vi "Win Receive data.vi"() -> ()   [LabVIEW 2017]
panel:
  in  "base path":path
  out "Waveform Chart":cluster{dbl, dbl, dbl}[](graph)
  out "error out":errorcluster
  in  "stop":bool
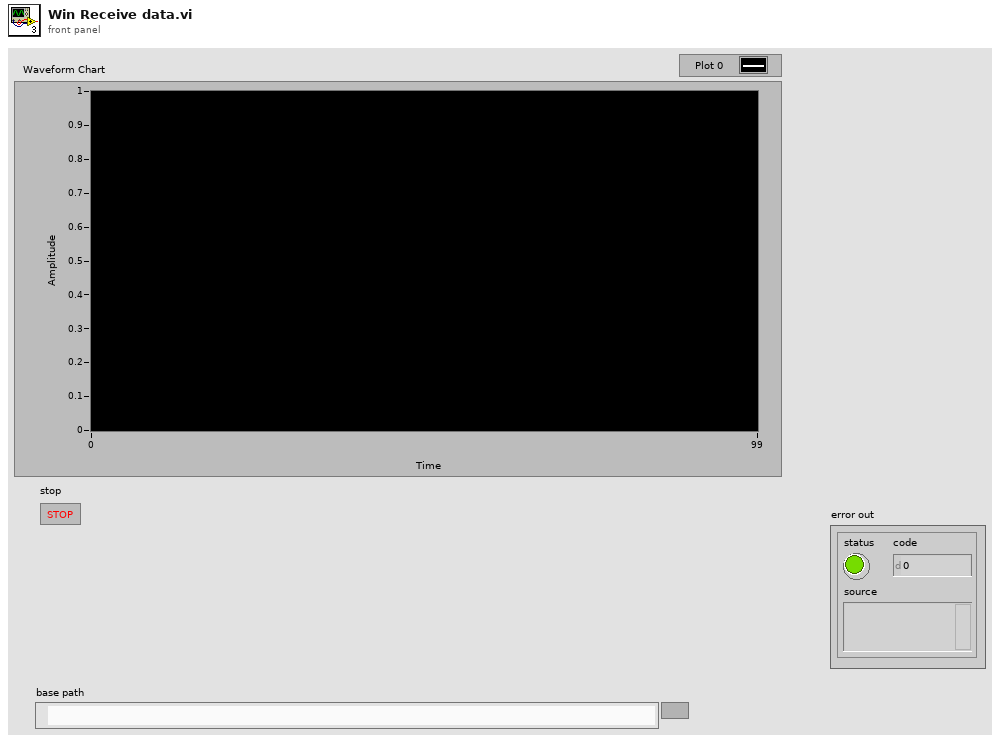
[diagram p1: front panel]
types:
  T1 = enum16{"open", "open or create", "create or replace", "create", "open (read-only)"}
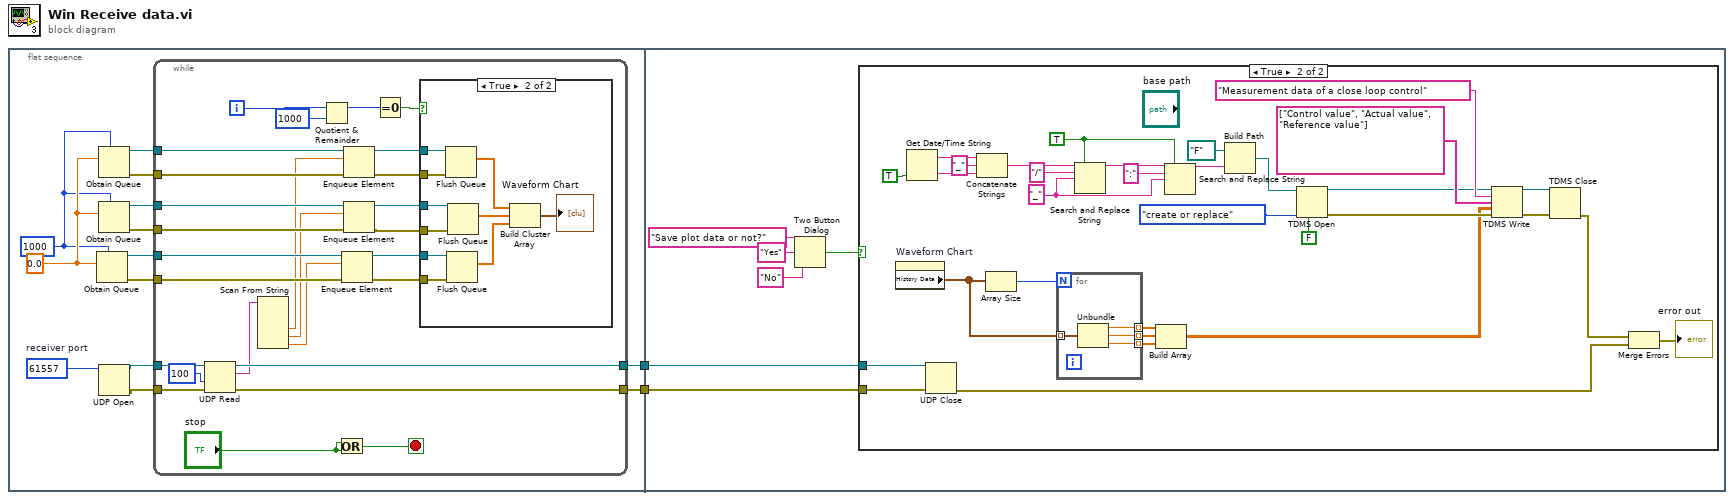
[diagram p0: block diagram]
diagram:
  n1 = flat-sequence {
    tunnel: [w4] -> w2
    tunnel: [w3] -> w1
    tunnel: w2 -> [w58]
    tunnel: w1 -> [w57]
    frame #0 {
      w12 = 0.0
      w11 = 1000 ("max queue size (-1, unlimited)")
      w15 = u16 61557  # receiver port
      n2 = Obtain Queue(max queue size (-1, unlimited)=w11, element data type=w12) -> (queue out=w6:refnum<queue>, error out=w5:errorcluster)  [unwired: 3 in, 1 out]
      n3 = Obtain Queue(max queue size (-1, unlimited)=w11, element data type=w12) -> (queue out=w10:refnum<queue>, error out=w9:errorcluster)  [unwired: 3 in, 1 out]
      n4 = Obtain Queue(max queue size (-1, unlimited)=w11, element data type=w12) -> (queue out=w8:refnum<queue>, error out=w7:errorcluster)  [unwired: 3 in, 1 out]
      n5 = UDP Open(11:w15) -> (port=w14:refnum<k16>, 0:w13:errorcluster)  [unwired: 4 in, 1 out]
      n6 = while {
        tunnel: w14 -> [w40]
        tunnel: w13 -> [w39]
        tunnel: w10 -> [w34]
        tunnel: w9 -> [w33]
        tunnel: w8 -> [w32]
        tunnel: w7 -> [w31]
        tunnel: w6 -> [w30]
        tunnel: w5 -> [w29]
        tunnel: [w22] -> w4
        tunnel: [w21] -> w3
        i -> [w36]
        stop <- w42 stop-if-true
        n7 = UDP Read(connection ID=w40, timeout ms (25000)=100 ("max size (548)"), 8:w39) -> (data out=w19:string, error out=w22:errorcluster, 3:w21:refnum<k16>)  [unwired: 3 out]
        n8 = Scan From String(input string=w19) -> (output 1=w16:dbl, output 2=w17:dbl, output 3=w18:dbl)  [unwired: 6 in, 3 out]
        n9 = Quotient & Remainder(x=w36, y=1000) -> (x-y*floor(x/y)=w37:i32)  [unwired: 1 out]
        n10 = Or(x="stop", y="stop") -> (x .or. y?=w42:bool)
        n11 = Enqueue Element(queue=w30, element=w18, error in (no error)=w29) -> (queue out=w24:refnum<queue>, error out=w23:errorcluster)  [unwired: 1 in, 1 out]
        n12 = Enqueue Element(queue=w34, element=w16, error in (no error)=w33) -> (queue out=w28:refnum<queue>, error out=w27:errorcluster)  [unwired: 1 in, 1 out]
        n13 = Enqueue Element(queue=w32, element=w17, error in (no error)=w31) -> (queue out=w26:refnum<queue>, error out=w25:errorcluster)  [unwired: 1 in, 1 out]
        n14 = Equal To 0?(x=w37) -> (x = 0?=w35:bool)
        n15 = case shown="True" w35 {
          tunnel: w28 -> [_ w49]
          tunnel: w27 -> [_ w48]
          tunnel: w26 -> [_ w47]
          tunnel: w25 -> [_ w46]
          tunnel: w24 -> [_ w45]
          tunnel: w23 -> [_ w44]
          frame False {
          }
          frame True {
            n16 = Flush Queue(queue=w49, error in (no error)=w48) -> (remaining elements=w51:dbl[])  [unwired: 2 out]
            n17 = Flush Queue(queue=w45, error in (no error)=w44) -> (remaining elements=w50:dbl[])  [unwired: 2 out]
            n18 = Flush Queue(queue=w47, error in (no error)=w46) -> (remaining elements=w52:dbl[])  [unwired: 2 out]
            n19 = Build Cluster Array(w51, w52, w50) -> (→"Waveform Chart":cluster{dbl, dbl, dbl}[])
          }
        }
      }
    }
    frame #1 {
      n20 = Two Button Dialog(message="Save plot data or not?", 1:"No" ("F button name (\"Cancel\")"), 2:"Yes" ("T button name (\"OK\")")) -> (T button?=w53:bool)
      n21 = case shown="True" w53 {
        tunnel: w58 -> [_ w90]
        tunnel: w57 -> [_ w89]
        frame False {
        }
        frame True {
          w68 = TRUE ("replace all? (F)")
          w69 = "_" ("replace string (\"\")")
          n22 = property on="Waveform Chart" class="WFChart (strict)"() -> ("History Data"=w61:cluster{dbl, dbl, dbl}[])  [unwired: 2 in, 2 out]
          n23 = Get Date/Time String(want seconds? (F)=TRUE) -> (date string=w67:string, time string=w74:string)  [unwired: 2 in]
          n24 = UDP Close(connection ID=w89, 8:w90) -> (error out=w64:errorcluster)  [unwired: 1 out]
          n25 = Concatenate Strings(w67, "_" ("string"), w74) -> (w73:string)
          n26 = Array Size(array=w61) -> (size(s)=w88:i32)
          n27 = for {
            N: w88 -> [_]
            tunnel: w61 -> [w94] mode=indexing
            tunnel: [w93] -> w87 mode=indexing
            tunnel: [w92] -> w86 mode=indexing
            tunnel: [w91] -> w85 mode=indexing
            n28 = Unbundle(w94) -> (w93:dbl, w92:dbl, w91:dbl)
          }
          n29 = Search and Replace String(replace all?=w68, input string=w73, search string="/", replace string=w69) -> (result string=w71:string)  [unwired: 4 in, 3 out]
          n30 = Build Array(w87, w86, w85) -> (w59:dbl[][])
          n31 = Search and Replace String(replace all?=w68, input string=w71, search string=":", replace string=w69) -> (result string=w65:string)  [unwired: 4 in, 3 out]
          n32 = Build Path(base path=path "F:/", name or relative path=w65) -> (appended path=w81:path)
          n33 = TDMS Open(6:FALSE ("disable buffering (T)"), 10:T1."create or replace" ("operation"), 11:w81) -> (0:w76:errorcluster, 3:w77:refnum<k34>)  [unwired: 4 in]
          n34 = TDMS Write(0:w77, 5:"Measurement data of a close loop control" ("group name in (Untitled)"), 7:string[] ["Control value", "Actual value", "Reference value"] ("channel names"), 9:w59, 11:w76) -> (4:w79:refnum<k34>, 15:w78:errorcluster)  [unwired: 1 in, 2 out]
          n35 = TDMS Close(8:w78, 11:w79) -> (0:w62:errorcluster)  [unwired: 1 out]
          n36 = Merge Errors(w62, w64) -> (→"error out":errorcluster)
        }
      }
    }
  }
